vi "FILO string.vi"(0 "Array":string[](array[string]), 2 "Array size":i32, 7 "String":string) -> (4 "Array out":string[](array[string]))   [LabVIEW 2014]
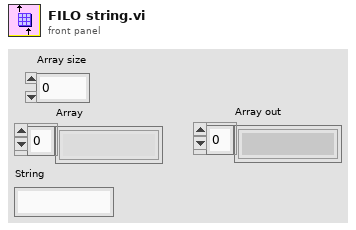
[diagram p1: front panel]
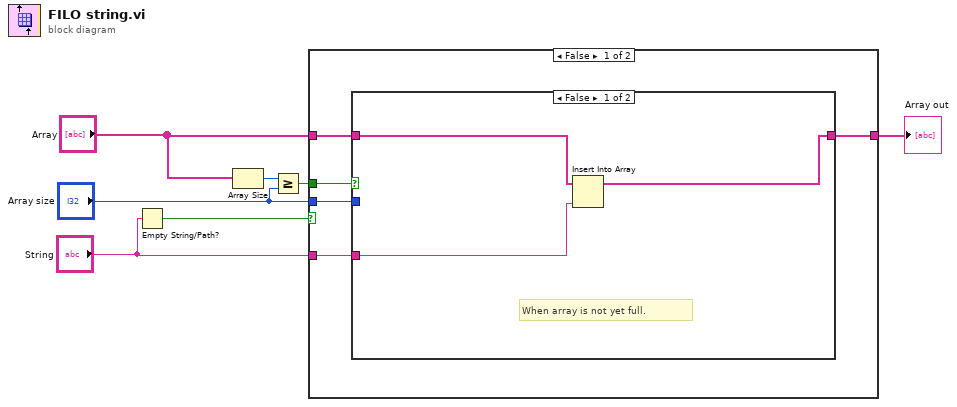
[diagram p0: block diagram]
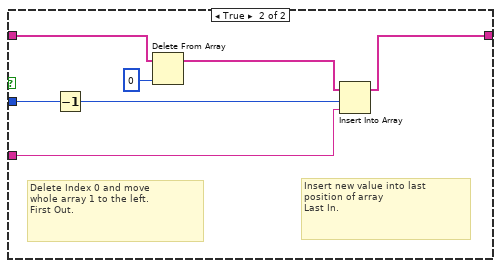
[diagram p2: hidden frame]
diagram:
  n1 = Empty String/Path?(string/path="String") -> (empty?=w1:bool)
  n2 = Array Size(array="Array") -> (size(s)=w7:i32)
  n3 = Greater Or Equal?(x=w7, y="Array size") -> (x >= y?=w6:bool)
  n4 = case shown="False" w1 {
    tunnel: w6 -> [w12 _]
    tunnel: "Array" -> [w11 w23]
    tunnel: "String" -> [w10 _]
    tunnel: [w9 w23] -> w4
    tunnel: "Array size" -> [w8 _]
    frame False {
      n5 = case shown="False" w12 {
        tunnel: [w13 w18] -> w9
        tunnel: w11 -> [w14 w21]
        tunnel: w10 -> [w15 w19]
        tunnel: w8 -> [_ w16]
        frame False {
          # "When array is not yet full."
          n6 = Insert Into Array(array=w14, new element=w15) -> (w13:string[])  [unwired: 1 in]
        }
        frame True {
          # "Insert new value into last\nposition of array\nLast In."
          # "Delete Index 0 and move \nwhole array 1 to the left.\nFirst Out."
          n7 = Decrement(x=w16) -> (x-1=w17:i32)
          n8 = Delete From Array(array=w21, index=0) -> (array with subset deleted=w20:string[])  [unwired: 1 in, 1 out]
          n9 = Insert Into Array(array=w20, index=w17, new element=w19) -> (w18:string[])
        }
      }
    }
    frame True {
      # "String is empty."
    }
  }
  "Array out" <- w4
